vi "resonant image correction.vi"(8 "shift index":i32(slide) scale=0.0..130.0, 10 "pixels per period (2pi, 2 lines)":dbl=1560.0, 11 "x pixels":i32=512) -> (2 "histogram cumsum":dbl[](graph), 3 "histogram pixels to avg":dbl[](graph))   [LabVIEW 2012]
uses:
  <vilib>/Analysis/NI_AALBase.lvlib
panel:
  out "histogram cumsum 2":dbl[](graph)
  out "Histogram: h(x)":i32[](array[numeric])
  out "Array":i32[](array[numeric])
  out "pixels per line":dbl
  out "Histogram Graph":T1(graph)
  out "Waveform Graph":dbl[](graph)
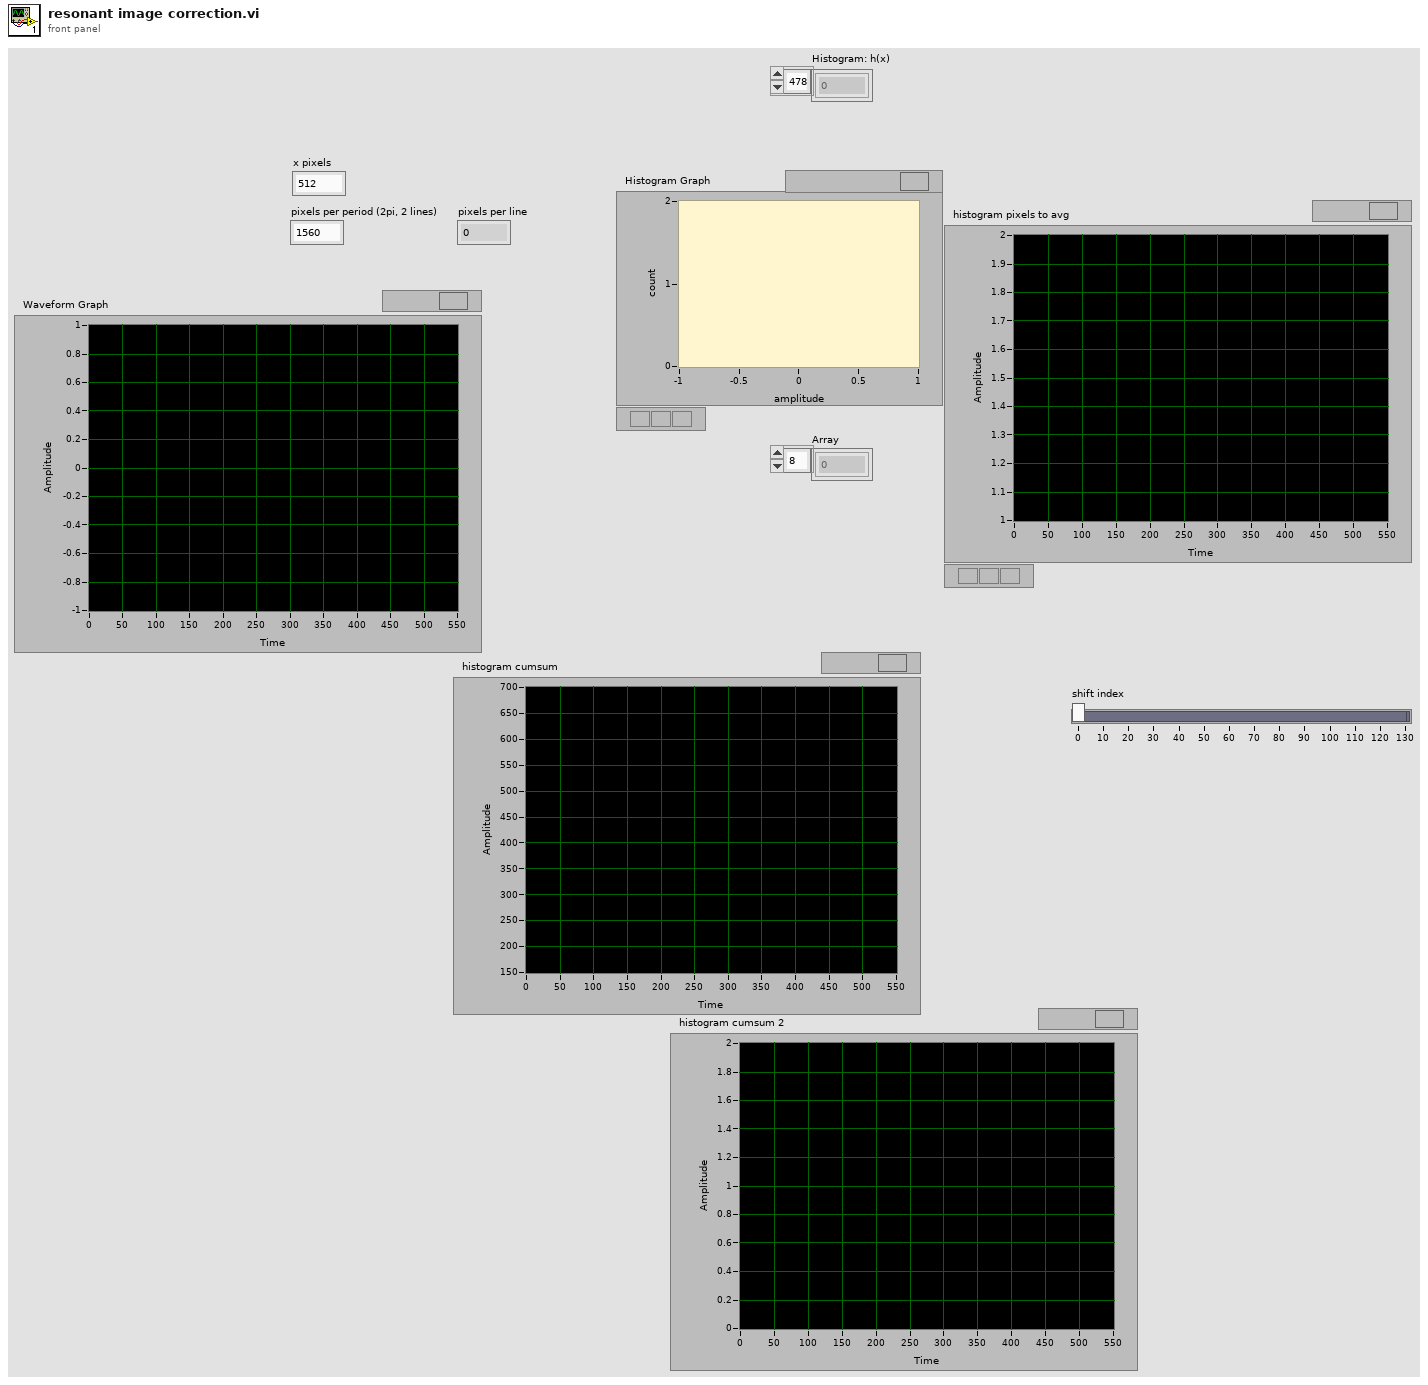
[diagram p1: front panel]
types:
  T1 = cluster{"X Values":dbl[], "Histogram: h(x)":i32[]}
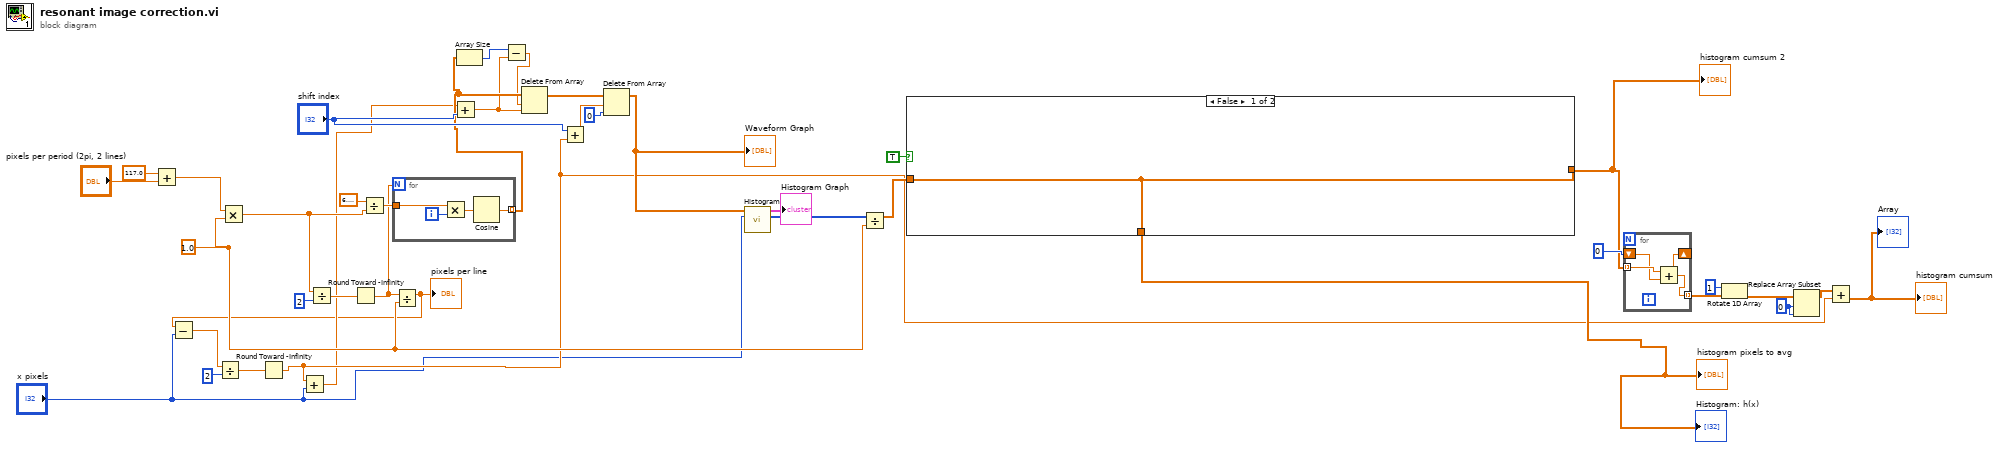
[diagram p0: block diagram]
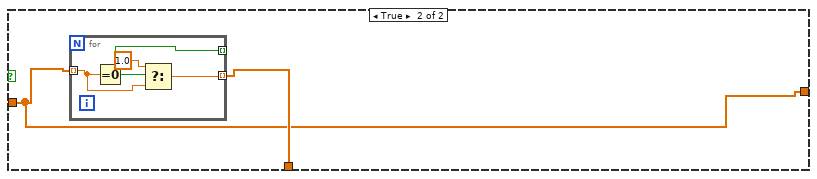
[diagram p2: hidden frame]
diagram:
  w26 = 1.0 ("y")
  w28 = 0 ("index")
  n1 = Add(x=117.0, y="pixels per period (2pi, 2 lines)") -> (x+y=w8:dbl)
  n2 = Multiply(x=w8, y=w26) -> (x*y=w27:dbl)
  n3 = Divide(x=w27, y=2 ("two lines per cycle")) -> (x/y=w36:dbl)
  n4 = Round Toward -Infinity(1:w36) -> (0:w33:dbl)
  n5 = Divide(x=6.283185307179586, y=w27) -> (x/y=w38:dbl)
  n6 = for {
    N: w33 -> [_]
    tunnel: w38 -> [w42]
    tunnel: [w40] -> w13 mode=indexing
    i -> [w41]
    n7 = Multiply(x=w42, y=w41) -> (x*y=w43:dbl)
    n8 = Cosine(x=w43) -> (cos(x)=w40:dbl)
  }
  n9 = Divide(x=w33, y=w26) -> (x/y=w1:dbl)
  "pixels per line" <- w1
  n10 = Subtract(x=w1, y="x pixels") -> (x-y=w5:dbl)
  n11 = Divide(x=w5, y=2 ("two lines per cycle")) -> (x/y=w6:dbl)
  n12 = Round Toward -Infinity(1:w6) -> (0:w4:dbl)
  n13 = Add(x=w4, y="x pixels") -> (x+y=w2:dbl)
  n14 = Add(x=w2, y="shift index") -> (x+y=w11:dbl)
  n15 = Array Size(array=w13) -> (size(s)=w12:i32)
  n16 = Subtract(x=w12, y=w11) -> (x-y=w10:dbl)
  n17 = Delete From Array(array=w13, length=w10, index=w11) -> (array with subset deleted=w18:dbl[])  [unwired: 1 out]
  n18 = Add(x="shift index", y=w4) -> (x+y=w22:dbl)
  n19 = Delete From Array(array=w18, length=w22, index=0 ("disabled index (col)")) -> (array with subset deleted=w17:dbl[])  [unwired: 1 out]
  "Waveform Graph" <- w17
  n20 = call <vilib>:"Histogram.vi"("intervals"="x pixels", "X"=w17) -> ("Histogram: h(x)"=w31:i32[], "Histogram Graph"=→"Histogram Graph":T1)  [unwired: 6 in, 2 out]
  n21 = Divide(x=w31, y=w26) -> (x/y=w24:dbl[])
  n22 = case shown="False" TRUE {
    tunnel: w24 -> [w44 w45]
    tunnel: [w44 w45] -> w14
    tunnel: [w44 w46] -> w16
    frame False {
    }
    frame True {
      n23 = for {
        tunnel: w45 -> [w49] mode=indexing
        tunnel: [w48] -> w46 mode=indexing
        tunnel: [w47] -> _ mode=indexing
        n24 = Equal To 0?(x=w49) -> (x = 0?=w47:bool)
        n25 = Select(t=1.0, s=w47, f=w49) -> (s? t:f=w48:dbl)
      }
    }
  }
  "histogram pixels to avg" <- w16
  "Histogram: h(x)" <- w16
  "histogram cumsum 2" <- w14
  n26 = for {
    tunnel: w14 -> [w53] mode=indexing
    shift-right: [w51] -> _
    shift-left: 0 -> [w52]
    tunnel: [w51] -> w32 mode=indexing
    n27 = Add(x=w53, y=w52) -> (x+y=w51:dbl)
  }
  n28 = Rotate 1D Array(1:w32, 2:1 ("n")) -> (0:w30:dbl[])
  n29 = Replace Array Subset(array=w30, new element=w28, index=w28) -> (w19:dbl[])
  n30 = Add(x=w19, y=w4) -> (x+y=→"histogram cumsum" →"Array":dbl[])
